vi "UpdateLanguage.vi"(8 "error in (no error)":errorcluster, 11 "Messages Actor in":refnum<class "Messages Actor.lvclass">) -> (0 "error out":errorcluster, 3 "Messages Actor out":refnum<class "Messages Actor.lvclass">)   [LabVIEW 2020, in "Messages Actor.lvlib" / "Messages Actor.lvclass"]
uses:
  Messages Actor.lvclass
  Messages Actor.lvclass/Messages Actor.ctl
  Read Language.vi
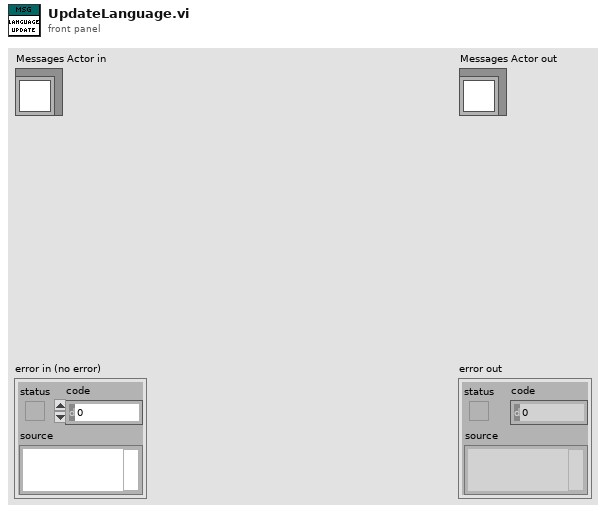
[diagram p1: front panel]
types:
  T1 = typedef "Language Enum.ctl" = enum16{"English", "Español", "Français"}
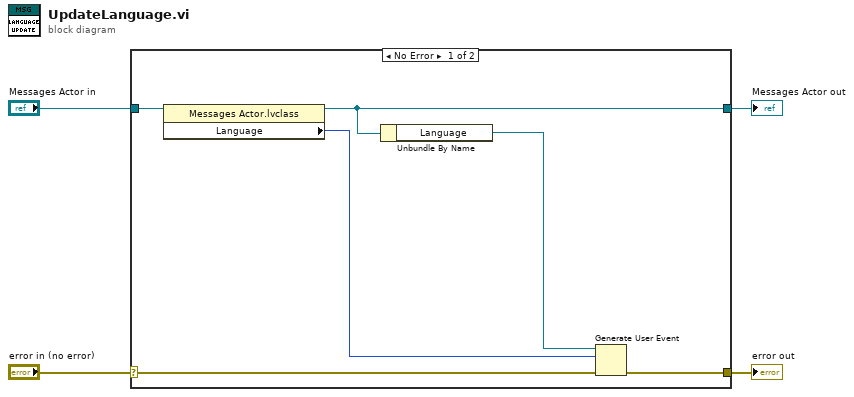
[diagram p0: block diagram]
diagram:
  n1 = case shown="No Error" "error in (no error)" {
    selector: "error in (no error)" -> [w9 w12]
    tunnel: [w8 w12] -> w3
    tunnel: [w7 w11] -> w1
    tunnel: "Messages Actor in" -> [w10 w11]
    frame No Error {
      n2 = property class="Messages Actor.lvclass"(reference=w10) -> (reference out=w7:refnum<class "Messages Actor.lvclass">, "Language"=w5:T1)  [unwired: 1 in, 1 out]
      n3 = Unbundle By Name(w7) -> ("Language"=w6:refnum<user-event>)
      n4 = Generate User Event(user event=w6, event data cluster=w5, error in=w9) -> (error out=w8:errorcluster)  [unwired: 1 in, 1 out]
    }
    frame Error {
    }
  }
  "error out" <- w3
  "Messages Actor out" <- w1
